vi "InputUpdate.vi"() -> ()   [LabVIEW 2016]
uses:
  <vilib>/Rock Robotics/WPI/Utilities/WPI_GetSetVariantRefNum.vi
  Globals/InputValues.vi
  <vilib>/Rock Robotics/Network Tables/NT Write Boolean Array.vi
  <vilib>/Rock Robotics/Network Tables/NT Write Numeric Array.vi
  Globals/Constantes.vi
panel:
  out "Triggers Combined Value":dbl
  in  "Use Triggers":bool
  out "OutputJoystick Y":dbl
  out "OutputJoystick X":dbl
  out "Joystick X":dbl
  out "Joystick Y":dbl
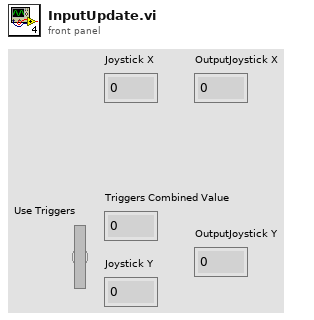
[diagram p1: front panel]
types:
  T1 = typedef "WPI_JoystickDevRef.ctl" = cluster{"Device":T2}
  T2 = typedef "WPI_JoystickDeviceEnum.ctl" = enum16{"USB 0", "USB 1", "USB 2", "USB 3", "USB 4", "USB 5"}
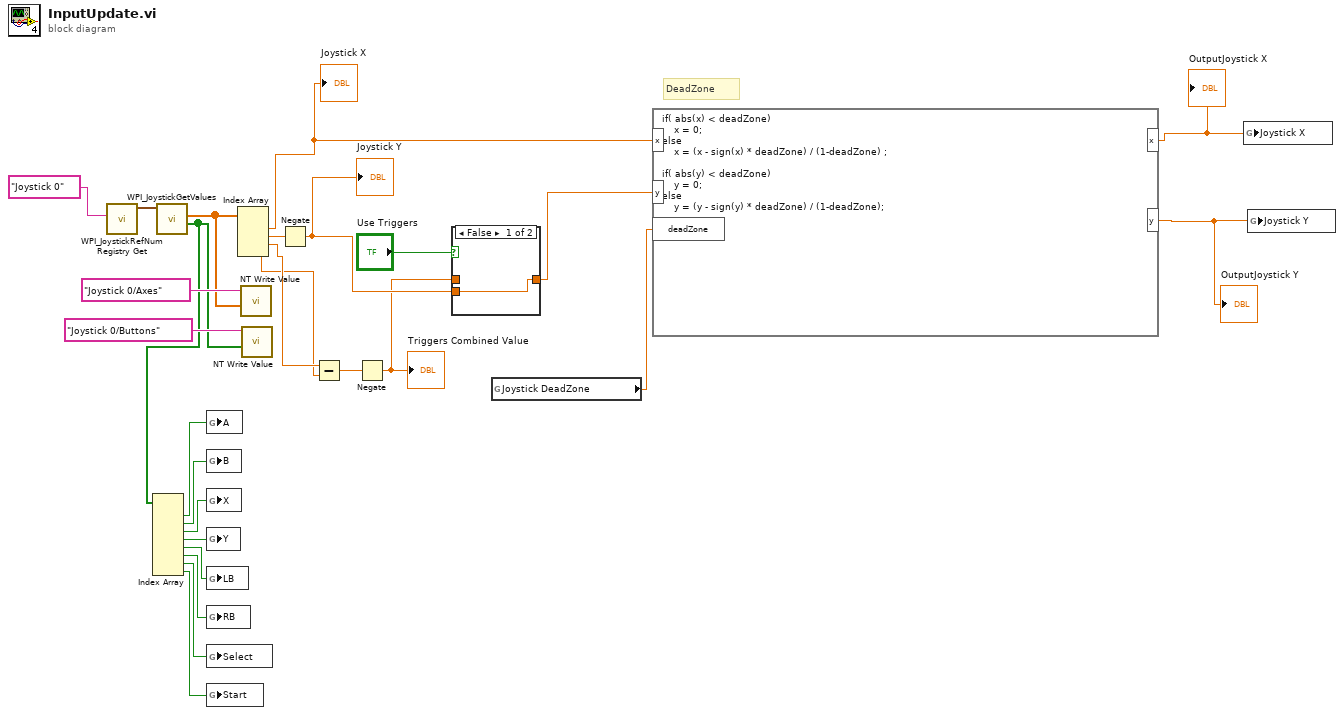
[diagram p0: block diagram]
diagram:
  # "DeadZone"
  n1 = call <vilib>:"WPI_JoystickRefNum Registry Get.vi"("refnum name"="Joystick 0") -> ("JoystickDevRef"=w25:T1)  [unwired: 1 in, 9 out]
  n2 = call <vilib>:"WPI_JoystickGetValues.vi"("JoystickDevRef"=w25) -> ("Buttons"=w9:bool[], "Axes"=w22:dbl[])  [unwired: 6 in, 3 out]
  n3 = Index Array(array=w9) -> (element #1=w8:bool, element #2=w7:bool, element #3=w6:bool, element #4=w5:bool, element #5=w4:bool, element #6=w3:bool, element #7=w2:bool, element #8=w1:bool)  [unwired: 8 in]
  n4 = global write "InputValues.vi" "A"(w8) -> ()
  n5 = global write "InputValues.vi" "B"(w7) -> ()
  n6 = global write "InputValues.vi" "X"(w6) -> ()
  n7 = global write "InputValues.vi" "Y"(w5) -> ()
  n8 = global write "InputValues.vi" "LB"(w4) -> ()
  n9 = global write "InputValues.vi" "RB"(w3) -> ()
  n10 = global write "InputValues.vi" "Select"(w2) -> ()
  n11 = global write "InputValues.vi" "Start"(w1) -> ()
  n12 = Index Array(array=w22) -> (element #1=w20:dbl, element #2=w16:dbl, element #3=w14:dbl, element #4=w10:dbl)  [unwired: 4 in]
  "Joystick X" <- w20
  n13 = call-poly <vilib>:"NT Write Value.vi"("Numeric Array"=w22, "Name"="Joystick 0/Axes") -> ()  [unwired: 9 in, 1 out]
  n14 = call-poly <vilib>:"NT Write Value.vi"("Boolean Array"=w9, "Name"="Joystick 0/Buttons") -> ()  [unwired: 9 in, 1 out]
  n15 = Negate(x=w16) -> (-x=w12:dbl)
  "Joystick Y" <- w12
  n16 = Subtract(x=w14, y=w10) -> (x-y=w15:dbl)
  n17 = Negate(x=w15) -> (-x=w11:dbl)
  "Triggers Combined Value" <- w11
  n18 = case shown="False" "Use Triggers" {
    tunnel: [w27 w28] -> w18
    tunnel: w12 -> [w27 _]
    tunnel: w11 -> [_ w28]
    frame False {
    }
    frame True {
    }
  }
  n19 = global read "Constantes.vi" "Joystick DeadZone"() -> (w21:dbl)
  n20 = formula code="if( abs(x) < deadZone)\n    x = 0;\nelse\n    x = (x - sign(x) * deadZone) / (1-deadZone) ;\n\nif( abs(y) < deadZone)\n    y = 0;\nelse\n    y = (y - sign(y) * deadZone) / (1-deadZone);"("y"=w18, "x"=w20, "deadZone"=w21) -> ("x"=w19:dbl, "y"=w13:dbl)
  "OutputJoystick X" <- w19
  "OutputJoystick Y" <- w13
  n21 = global write "InputValues.vi" "Joystick X"(w19) -> ()
  n22 = global write "InputValues.vi" "Joystick Y"(w13) -> ()
